vi "FindBaseAndNearestImplementations.vi"(8 "error in (no error)":errorcluster, 10 "Method Name":string, 11 "LVClassLibrary in":refnum<vi>) -> (0 "error out":errorcluster, 1 "Opened Refs":refnum<vi>[](array[refnum]), 2 "Nearest Implementation":refnum<vi>, 3 "Base Implementation":refnum<vi>)   [LabVIEW 2017, in "DynamicDispatchImplementationWalker.lvlib"]
uses:
  DynamicDispatchImplementationWalker.lvlib
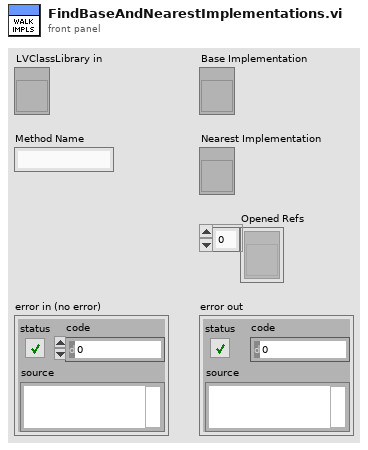
[diagram p1: front panel]
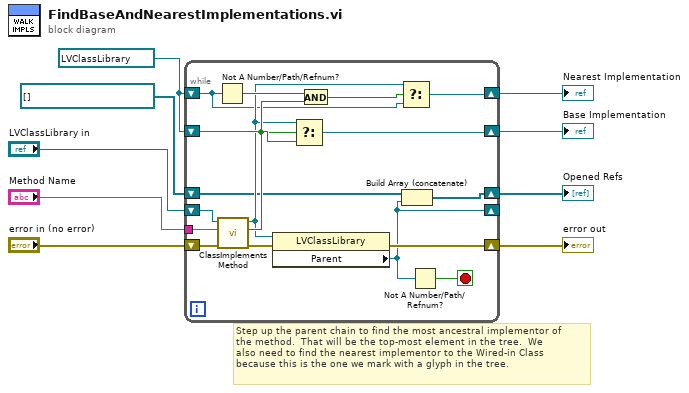
[diagram p0: block diagram]
diagram:
  w6 = refnum<vi> refnum ("Class Refnum out")
  # "Step up the parent chain to find the most ancestral implementor of\nthe method.  That will be the top-most element in the tree.  We\nalso need to find the nearest implementor to the Wired-in Class\nbecause this is the one we mark with a glyph in the tree."
  n1 = while {
    shift-right: [w20] -> w1
    shift-left: w6 -> [w21]
    shift-right: [w12] -> _
    shift-left: "LVClassLibrary in" -> [w24]
    shift-right: [w13] -> w3
    shift-left: "error in (no error)" -> [w25]
    tunnel: "Method Name" -> [w23]
    shift-right: [w14] -> w2
    shift-left: w6 -> [w15]
    shift-right: [w10] -> w8
    shift-left: refnum<vi>[] [] -> [w11]
    stop <- w26 stop-if-true
    n2 = Not A Number/Path/Refnum?(number/path/refnum=w15) -> (NaN/Path/Refnum?=w19:bool)
    n3 = call "ClassImplementsMethod.vi"("error in (no error)"=w25, "Method Name"=w23, "Class Refnum"=w24) -> ("error out"=w22:errorcluster, "Implements method?"=w18:bool, "Class Refnum out"=w16:refnum<vi>)  [unwired: 5 in, 1 out]
    n4 = property class="LVClassLibrary"(reference=w16, error in=w22) -> (error out=w13:errorcluster, "Parent"=w12:refnum<vi>)  [unwired: 1 out]
    n5 = Select(t=w16, s=w18, f=w21) -> (s? t:f=w20:refnum<vi>)
    n6 = And(x=w19, y=w18) -> (x .and. y?=w17:bool)
    n7 = Select(t=w16, s=w17, f=w15) -> (s? t:f=w14:refnum<vi>)
    n8 = Build Array (concatenate)(w11, w12) -> (w10:refnum<vi>[])
    n9 = Not A Number/Path/Refnum?(number/path/refnum=w12) -> (NaN/Path/Refnum?=w26:bool)
  }
  "Opened Refs" <- w8
  "Base Implementation" <- w1
  "error out" <- w3
  "Nearest Implementation" <- w2
